vi "Validate Hardware Custom Device.vi"(8 "error in (no error)":errorcluster, 11 "Hardware Ref in":T1 format="%.0x") -> (0 "error out":errorcluster, 3 "Hardware Ref out":T1 format="%.0x")   [LabVIEW 2017, in "Routing and Faulting Hardware API.lvlib"]
uses:
  Routing and Faulting Hardware API.lvlib
  <vilib>/NI Veristand/Custom Device API/Custom Device Item Ref.ctl
  <vilib>/NI Veristand/Custom Device API/Custom Device API.lvlib
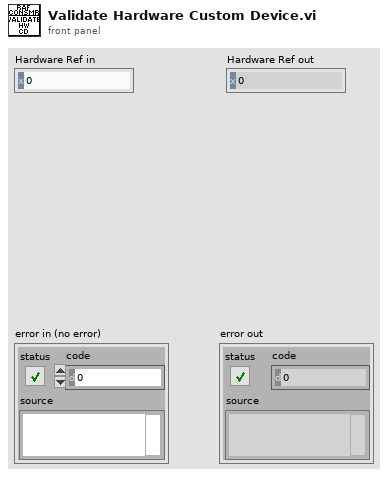
[diagram p1: front panel]
types:
  T1 = typedef "Custom Device API.lvlib/Custom Device Item Ref.ctl" = u64
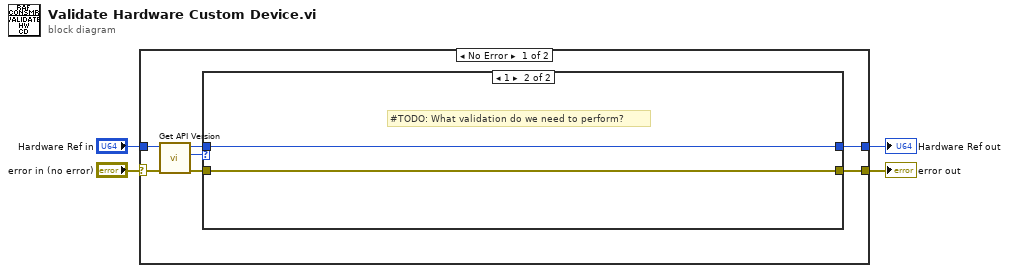
[diagram p0: block diagram]
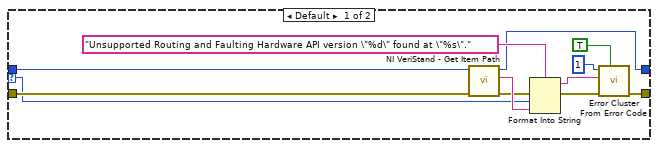
[diagram p2: hidden frame]
diagram:
  n1 = case shown="No Error" "error in (no error)" {
    selector: "error in (no error)" -> [w10 w27]
    tunnel: [w9 w27] -> w3
    tunnel: [w5 w26] -> w2
    tunnel: "Hardware Ref in" -> [w11 w26]
    frame No Error {
      n2 = call "Get API Version.vi"("error in (no error)"=w10, "Hardware Ref in"=w11) -> ("error out"=w8:errorcluster, "API version"=w6:i32, "Hardware Ref out"=w7:T1)  [unwired: 7 in]
      n3 = case shown="1" w6 {
        selector: w6 -> [w13 _]
        tunnel: [w23 w24] -> w9
        tunnel: w8 -> [w20 w24]
        tunnel: w7 -> [w19 w25]
        tunnel: [w12 w25] -> w5
        frame Default {
          n4 = call <vilib>:"NI VeriStand - Get Item Path.vi"("error in (no error)"=w20, "Item Ref in"=w19) -> ("error out"=w15:errorcluster, "Path"=w17:string, "Item Ref out"=w12:T1)  [unwired: 6 in, 1 out]
          n5 = Format Into String(format string="Unsupported Routing and Faulting Hardware API version \"%d\" found at \"%s\"." ("error message (\"\")"), error in=w15, w13, w17) -> (resulting string=w14:string, error out=w16:errorcluster)  [unwired: 1 in]
          n6 = call <vilib>:"Error Cluster From Error Code.vi"("show call chain? (False)"=TRUE, "error in (no error)"=w16, "error message (\"\")"=w14, "error code (0)"=1) -> ("error out"=w23:errorcluster)  [unwired: 5 in]
        }
        frame 1 {
          # "#TODO: What validation do we need to perform?"
        }
      }
    }
    frame Error {
    }
  }
  "error out" <- w3
  "Hardware Ref out" <- w2
